vi "Tune Jaguar PID.vi"() -> ()   [LabVIEW 2011]
uses:
  <vilib>/Rock Robotics/WPI/CAN/Jaguar/SubVIs/WPI_CANJaguar_StatusSelect.ctl
panel:
  out "Shooter 2 Speed":dbl
  out "Shooter 1 Speed":dbl
  in  "Motor Speed":dbl
  in  "P":dbl
  in  "I":dbl
  in  "D":dbl
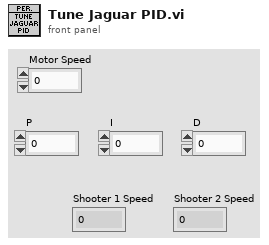
[diagram p1: front panel]
types:
  T1 = typedef "WPI_CANJaguar_StatusSelect.ctl" = enum16{"Output Percent VBus", "Output Voltage", "Bus Voltage", "Current", "Temperature", "Position", "Speed", "Limit Switches", "Faults", "Fault Counters", "Power Cycle"}
  T2 = typedef "WPI_JoystickDevRef.ctl" = cluster{"Device":T3}
  T3 = typedef "WPI_JoystickDeviceEnum.ctl" = enum16{"USB 1", "USB 2", "USB 3", "USB 4", "Kinect 1", "Kinect 2"}
  T4 = cluster{"axis 1 (x)":dbl, "axis 2 (y)":dbl, "axis 3 (throttle)":dbl, "axis 4":dbl, "axis 5":dbl, "axis 6":dbl}
  T5 = typedef "WPI_MotorControlDeviceRef.ctl" = cluster{"DeviceStatus":errorcluster, "Type":enum16{"PWM", "CAN"}, "PWM":cluster{"Digital Module":T6, "PWM Channel":T7, "DeadBand":T8}, "CAN":cluster{"Device Number":u8, "Control Mode":T9, "Semaphore":T10, "Max Vout":dbl}, "Invert":bool, "TransformRef":T11, "InvTransformRef":T11}
  T6 = typedef "FPGA_TypedefDigitalModule.ctl" = enum16{"Digital Module 1", "Digital Module 2"}
  T7 = typedef "FPGA_DIOPWMChannel.ctl" = enum8{"PWM 1", "PWM 2", "PWM 3", "PWM 4", "PWM 5", "PWM 6", "PWM 7", "PWM 8", "PWM 9", "PWM 10", "Invalid"}
  T8 = typedef "WPI_PWMDeadband.ctl" = cluster{"Name":string, "maxPositivePwm":i32, "minPositivePwm":i32, "centerPwm":i32, "maxNegativePwm":i32, "minNegativePwm":i32, "angularRange":u16}
  T9 = typedef "WPI_CANJaguar_ControlMode.ctl" = enum8{"Percent VBus", "Current", "Speed", "Position", "Voltage"}
  T10 = typedef "Semaphore RefNum" = refnum<k1>
  T11 = typedef "WPI_PWMTransform_ConPane.ctl" = refnum<vi>
  T12 = typedef "WPI_CANJaguar_Status.ctl" = cluster{"Output Percent VBus":dbl, "Output Voltage":dbl, "Bus Voltage":dbl, "Current":dbl, "Temperature":dbl, "Position":dbl, "Speed":dbl, "Limits":cluster{"Forward Limit":bool, "Reverse Limit":bool, "Forward Soft Limit":bool, "Reverse Soft Limit":bool, "Sticky Forward Limit":bool, "Sticky Reverse Limit":bool, "Sticky Forward Soft Limit":bool, "Sticky Reverse Soft Limit":bool}, "Faults":cluster{"Current Fault":bool, "Temperature Fault":bool, "Bus Voltage Fault":bool, "Gate Driver Fault":bool, "Comm Fault":bool}, "Fault Counters":cluster{"Current Faults":u8, "Temperature Faults":u8, "Bus Voltage Faults":u8, "Gate Driver Faults":u8, "Comm Faults":u8, "CAN Status":u8, "CAN RX Errors":u8, "CAN TX Errors":u8}, "Power Cycle":bool}
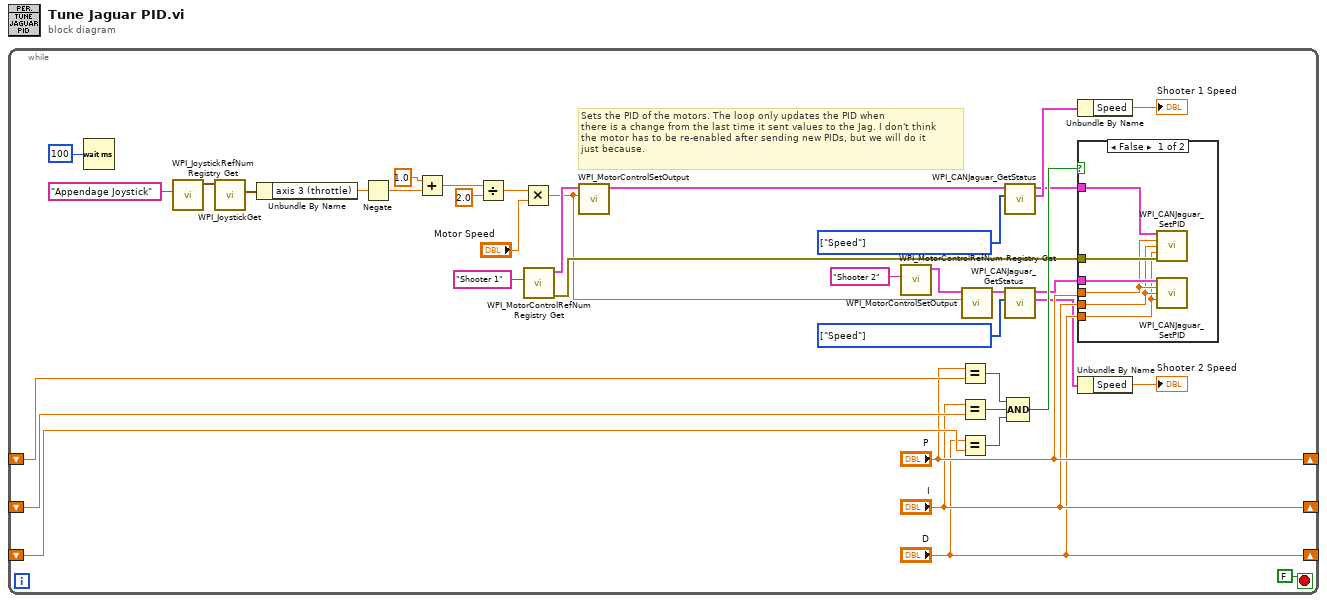
[diagram p0: block diagram]
diagram:
  n1 = while {
    shift-right: ["P"] -> _
    shift-left: _ -> [w36]
    shift-right: ["I"] -> _
    shift-left: _ -> [w34]
    shift-right: ["D"] -> _
    shift-left: _ -> [w30]
    stop <- FALSE stop-if-true
    w15 = T1[] [enum."Speed"] items=["Output Percent VBus", "Output Voltage", "Bus Voltage", "Current", "Temperature", "Position", "Speed", "Limit Switches", "Faults", "Fault Counters", "Power Cycle"] ("Status Select")
    w20 = T1[] [enum."Speed"] items=["Output Percent VBus", "Output Voltage", "Bus Voltage", "Current", "Temperature", "Position", "Speed", "Limit Switches", "Faults", "Fault Counters", "Power Cycle"] ("Status Select")
    # "Sets the PID of the motors. The loop only updates the PID when\nthere is a change from the last time it sent values to the Jag. I don't think\nthe motor has to be re-enabled after sending new PIDs, but we will do it\njust because."
    n2 = Wait (ms)(milliseconds to wait=u32 100) -> ()  [unwired: 1 out]
    n3 = call <vilib>:"WPI_JoystickRefNum Registry Get.vi"("refnum name"="Appendage Joystick") -> ("JoystickDevRef"=w10:T2)  [unwired: 9 in, 1 out]
    n4 = call <vilib>:"WPI_JoystickGet.vi"("JoystickDevRef"=w10) -> ("Axes"=w9:T4)  [unwired: 4 in, 2 out]
    n5 = Unbundle By Name(w9) -> ("axis 3 (throttle)"=w8:dbl)
    n6 = Negate(x=w8) -> (-x=w7:dbl)
    n7 = Add(x=1.0, y=w7) -> (x+y=w5:dbl)
    n8 = Divide(x=w5, y=2.0) -> (x/y=w3:dbl)
    n9 = Multiply(x=w3, y="Motor Speed") -> (x*y=w1:dbl)
    n10 = call <vilib>:"WPI_MotorControlRefNum Registry Get.vi"("refnum name"="Shooter 1") -> ("error out"=w24:errorcluster, "MotorControlDevRef"=w25:T5)  [unwired: 9 in]
    n11 = call <vilib>:"WPI_MotorControlSetOutput.vi"("Output"=w1, "MotorControlDevRef"=w25) -> ("MotorControlDevRef"=w18:T5)  [unwired: 8 in, 1 out]
    n12 = call <vilib>:"WPI_MotorControlRefNum Registry Get.vi"("refnum name"="Shooter 2") -> ("MotorControlDevRef"=w22:T5)  [unwired: 9 in, 1 out]
    n13 = Equal?(x="P", y=w36) -> (x = y?=w35:bool)
    n14 = Equal?(x="I", y=w34) -> (x = y?=w33:bool)
    n15 = Equal?(x="D", y=w30) -> (x = y?=w32:bool)
    n16 = call <vilib>:"WPI_MotorControlSetOutput.vi"("Output"=w1, "MotorControlDevRef"=w22) -> ("MotorControlDevRef"=w13:T5)  [unwired: 8 in, 1 out]
    n17 = call <vilib>:"WPI_CANJaguar_GetStatus.vi"("Status Select"=w20, "CAN Jaguar Ref"=w18) -> ("Status"=w21:T12, "CAN Jaguar Ref Out"=w17:T5)  [unwired: 7 in, 1 out]
    n18 = call <vilib>:"WPI_CANJaguar_GetStatus.vi"("Status Select"=w15, "CAN Jaguar Ref"=w13) -> ("Status"=w16:T12, "CAN Jaguar Ref Out"=w12:T5)  [unwired: 7 in, 1 out]
    n19 = Compound Arithmetic op=AND(w35, w33, w32) -> (w31:bool)
    n20 = Unbundle By Name(w21) -> ("Speed"=→"Shooter 1 Speed":dbl)
    n21 = case shown="False" w31 {
      tunnel: "P" -> [w41 _]
      tunnel: "I" -> [w40 _]
      tunnel: "D" -> [w39 _]
      tunnel: w17 -> [w44 _]
      tunnel: w24 -> [w43 _]
      tunnel: w12 -> [w42 _]
      frame False {
        n22 = call <vilib>:"WPI_CANJaguar_SetPID.vi"("CAN Jaguar Ref"=w44, "P"=w41, "I"=w40, "D"=w39, "error in (no error)"=w43) -> ()  [unwired: 9 in, 2 out]
        n23 = call <vilib>:"WPI_CANJaguar_SetPID.vi"("CAN Jaguar Ref"=w42, "P"=w41, "I"=w40, "D"=w39) -> ()  [unwired: 10 in, 2 out]
      }
      frame True {
      }
    }
    n24 = Unbundle By Name(w16) -> ("Speed"=→"Shooter 2 Speed":dbl)
  }
